vi "Ready to Log.vi"(8 "error in (no error)":errorcluster, 10 "UUID":string, 11 "CubeLogger in":refnum<class "CubeLogger.lvclass">) -> (0 "error out":errorcluster, 2 "Ready?":bool, 3 "CubeLogger out":refnum<class "CubeLogger.lvclass">)   [LabVIEW 2018, in "CubeLogger.lvclass"]
uses:
  CubeLogger.lvclass
  CubeLogger.lvclass/CubeLogger.ctl
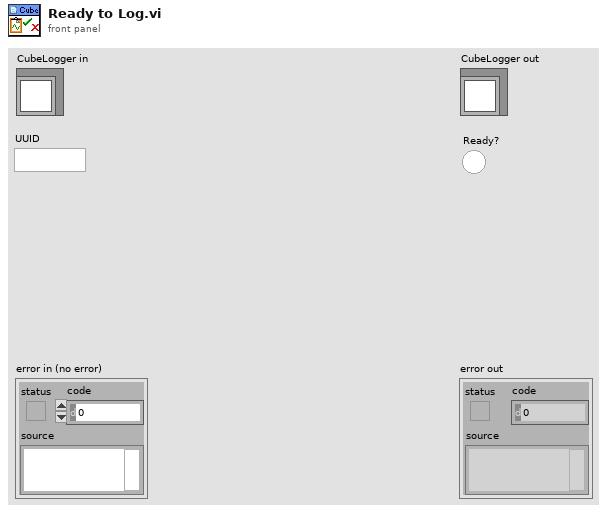
[diagram p1: front panel]
types:
  T1 = typedef "CubeLogger.lvclass/Dataset.ctl" = cluster{"name":string, "path":string, "size":i32[], "type":enum16{"single", "double", "uint8", "uint16", "uint32", "uint64", "int8", "int16", "int32", "int64"}, "mfmt":string}
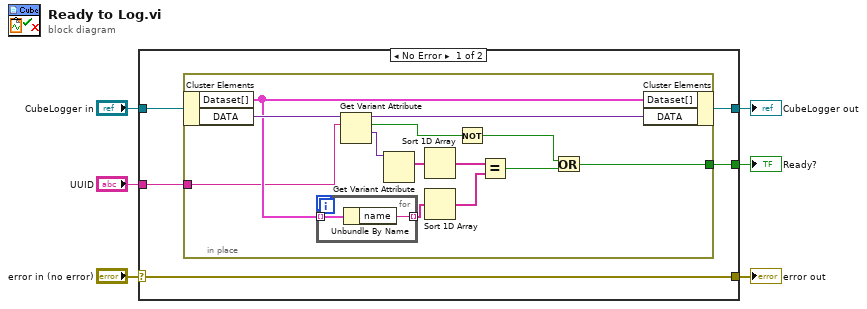
[diagram p0: block diagram]
diagram:
  n1 = case shown="No Error" "error in (no error)" {
    selector: "error in (no error)" -> [w11 w28]
    tunnel: [w11 w28] -> w5
    tunnel: [w10 w27] -> w3
    tunnel: "CubeLogger in" -> [w9 w27]
    tunnel: "UUID" -> [w8 _]
    tunnel: [w7 _] -> w1
    frame No Error {
      n2 = in-place {
        in-place-border: [w15] -> w7
        in-place-border: w8 -> [w18]
        n3 = in-place-cluster #1(w9) -> ("Dataset[]"=w23:T1[], "DATA"=w24:variant)
        n4 = for {
          tunnel: w23 -> [w26] mode=indexing
          tunnel: [w25] -> w22 mode=indexing
          n5 = Unbundle By Name(w26) -> ("name"=w25:string)
        }
        n6 = Get Variant Attribute(Variant=w24, name=w18) -> (duplicate Variant=w14:variant, found=w13:bool, value=w17:variant)  [unwired: 2 in, 1 out]
        n7 = Get Variant Attribute(Variant=w17) -> (names=w21:string[])  [unwired: 3 in, 3 out]
        n8 = Sort 1D Array(array=w21) -> (sorted array=w20:string[])
        n9 = Sort 1D Array(array=w22) -> (sorted array=w19:string[])
        n10 = Not(x=w13) -> (.not. x?=w12:bool)
        n11 = Equal?(x=w20, y=w19) -> (x = y?=w16:bool)
        n12 = Or(x=w12, y=w16) -> (x .or. y?=w15:bool)
        n13 = in-place-cluster #1("Dataset[]"=w23, "DATA"=w14) -> (w10:refnum<class "CubeLogger.lvclass">)
      }
    }
    frame Error {
    }
  }
  "error out" <- w5
  "CubeLogger out" <- w3
  "Ready?" <- w1
